vi "数据写入database.vi"(9 "data输入":T2) -> (1 "error out":errorcluster)   [LabVIEW 2016, in "斯坦道CODMn.lvlib"]
uses:
  <vilib>/Utility/error.llb/DialogType.ctl
panel:
  out "输出簇":T1
  in  "error in (no error)":errorcluster
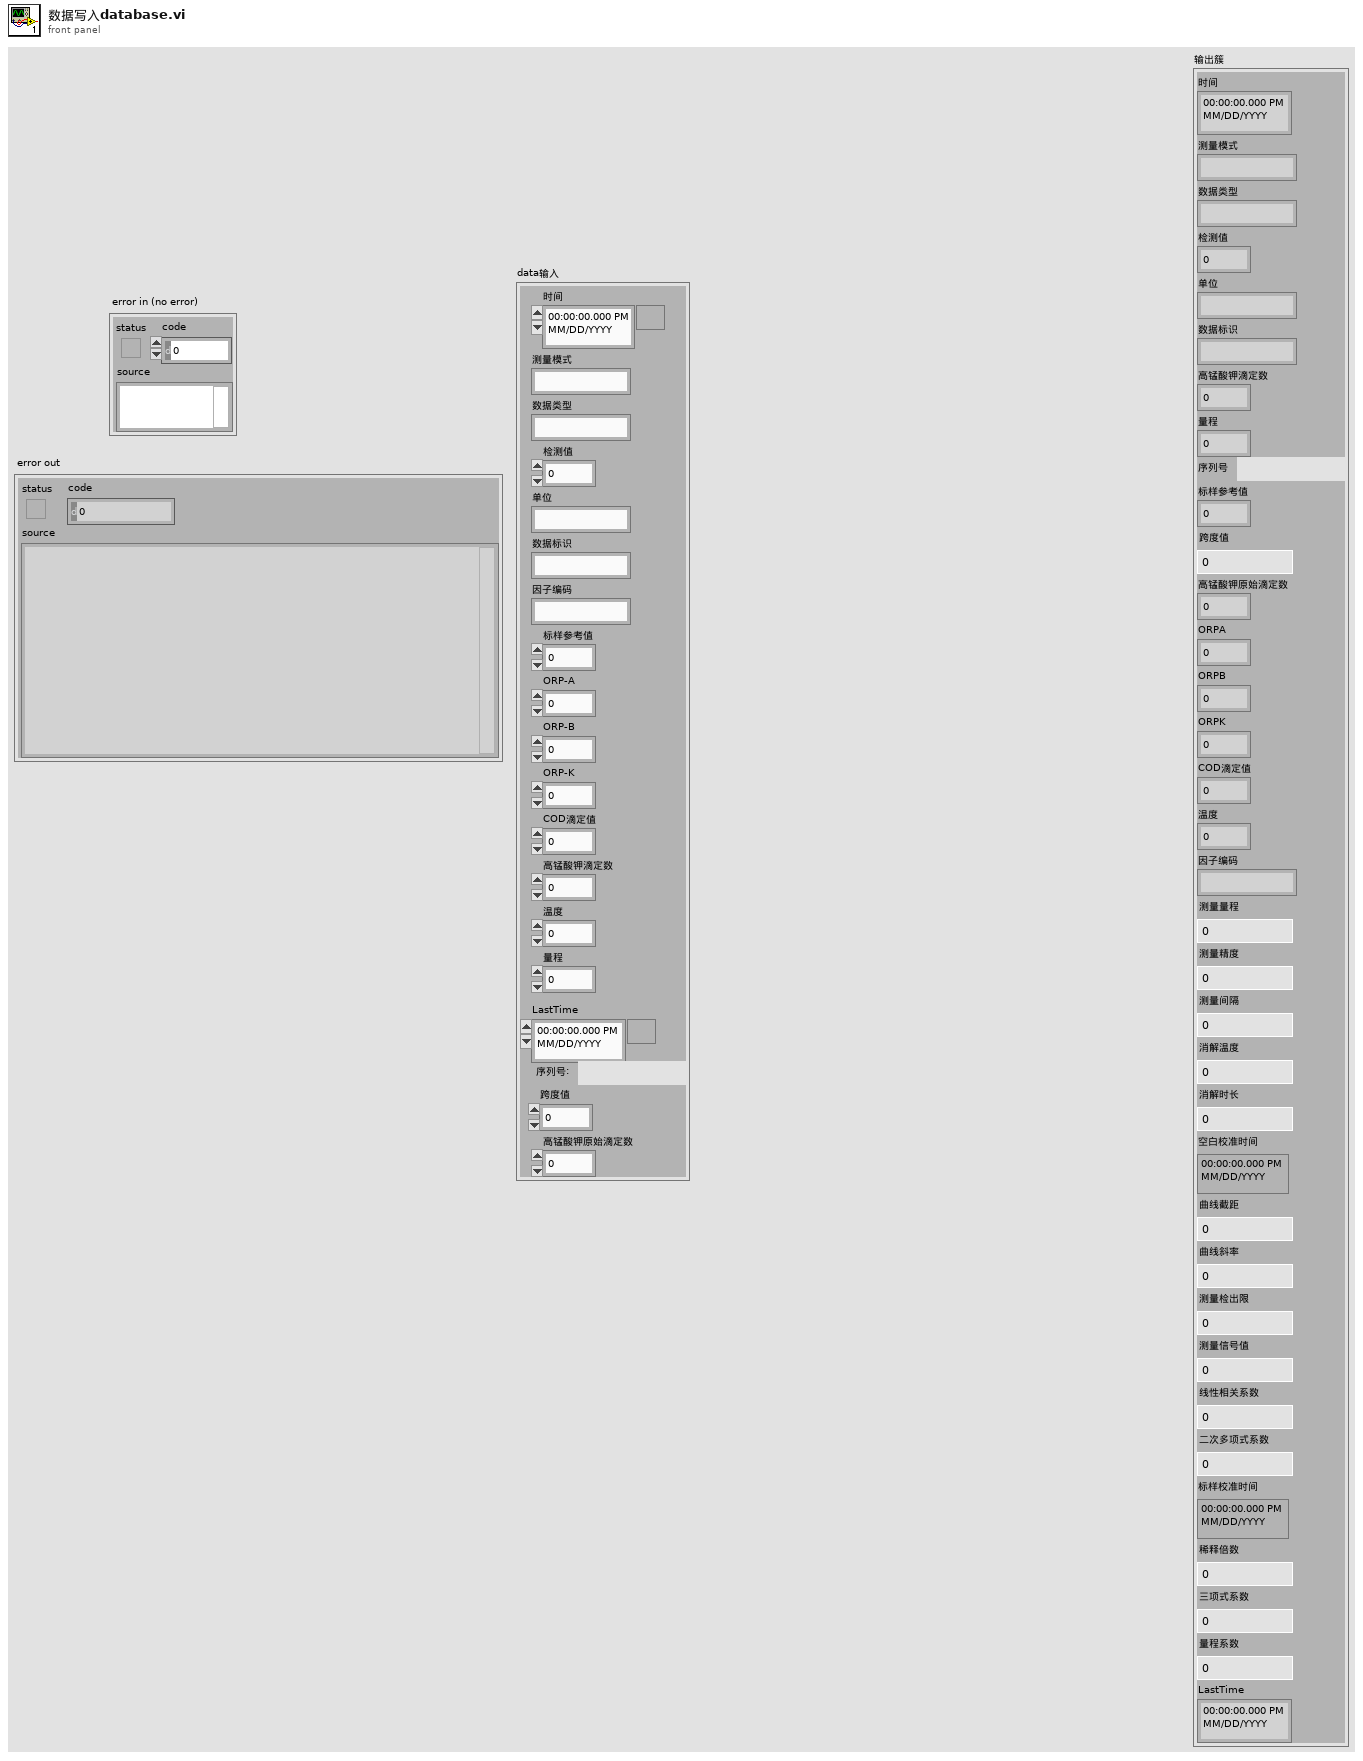
[diagram p1: front panel]
types:
  T1 = typedef "PLC版 CODMn字段定义.ctl" = cluster{"时间":timestamp, "测量模式":string, "数据类型":string, "检测值":sgl, "单位":string, "数据标识":string, "高锰酸钾滴定数":sgl, "量程":sgl, "序列号":string, "标样参考值":sgl, "跨度值":sgl, "高锰酸钾原始滴定数":sgl, "ORPA":sgl, "ORPB":sgl, "ORPK":sgl, "COD滴定值":sgl, "温度":sgl, "因子编码":string, "测量量程":sgl, "测量精度":sgl, "测量间隔":sgl, "消解温度":sgl, "消解时长":sgl, "空白校准时间":timestamp, "曲线截距":sgl, "曲线斜率":sgl, "测量检出限":sgl, "测量信号值":sgl, "线性相关系数":sgl, "二次多项式系数":sgl, "标样校准时间":timestamp, "稀释倍数":sgl, "三项式系数":sgl, "量程系数":sgl, "LastTime":timestamp}
  T2 = cluster{"时间":timestamp, "测量模式":string, "数据类型":string, "检测值":sgl, "单位":string, "数据标识":string, "因子编码":string, "标样参考值":sgl, "ORP-A":sgl, "ORP-B":sgl, "ORP-K":sgl, "COD滴定值":sgl, "高锰酸钾滴定数":sgl, "温度":sgl, "量程":sgl, "LastTime":timestamp, "序列号:":string, "跨度值":sgl, "高锰酸钾原始滴定数":sgl}
  T3 = typedef "DialogType.ctl" = u16
  T4 = cluster{"测量量程":dbl, "测量精度":dbl, "测量间隔":dbl, "消解温度":dbl, "消解时长":dbl, "空白校准时间":timestamp, "曲线截距":dbl, "曲线斜率":dbl, "测量检出限":dbl, "测量信号值":dbl, "线性相关系数":dbl, "二次多项式系数":dbl, "标样校准时间":timestamp, "稀释倍数":dbl, "三项式系数":dbl, "空白标定系数":dbl, "量程系数":dbl, "F0/ORPA":dbl, "F1/ORPB":dbl, "F2/ORPK":dbl, "F3":dbl, "F4":dbl, "F5":dbl, "F6":dbl, "F7":dbl, "X0/滴定数":dbl, "量程":dbl}
  T5 = typedef "数据库类型.ctl" = enum16{"Access", "SQLite"}
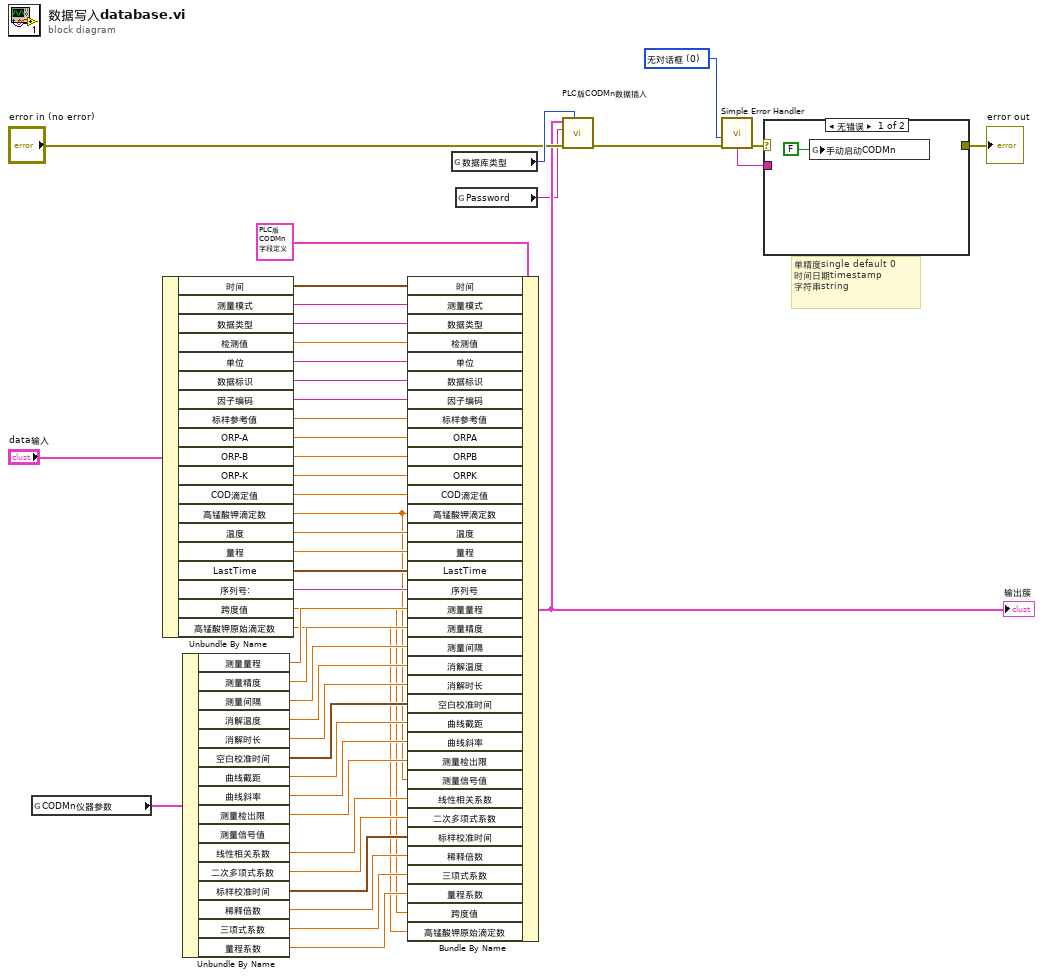
[diagram p0: block diagram]
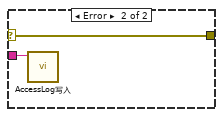
[diagram p2: hidden frame]
diagram:
  w46 = T3 0 items=["无对话框", "确定信息", "继续或停止信息", "确定信息＋警告", "继续/停止+警告"] ("type of dialog (OK msg:1)")
  # "单精度single default 0\n时间日期timestamp\n字符串string"
  n1 = global read "CODMn断电保存全局变量.vi" "CODMn仪器参数"() -> (w25:T4)
  n2 = Unbundle By Name("data输入") -> ("时间"=w41:timestamp, "测量模式"=w40:string, "数据类型"=w39:string, "检测值"=w38:sgl, "单位"=w37:string, "数据标识"=w36:string, "因子编码"=w35:string, "标样参考值"=w34:sgl, "ORP-A"=w33:sgl, "ORP-B"=w32:sgl, "ORP-K"=w31:sgl, "COD滴定值"=w30:sgl, "高锰酸钾滴定数"=w8:sgl, "温度"=w29:sgl, "量程"=w28:sgl, "LastTime"=w27:timestamp, "序列号:"=w26:string, "跨度值"=w9:sgl, "高锰酸钾原始滴定数"=w2:sgl)
  n3 = Unbundle By Name(w25) -> ("测量量程"=w24:dbl, "测量精度"=w23:dbl, "测量间隔"=w22:dbl, "消解温度"=w21:dbl, "消解时长"=w20:dbl, "空白校准时间"=w19:timestamp, "曲线截距"=w18:dbl, "曲线斜率"=w17:dbl, "测量检出限"=w16:dbl, "线性相关系数"=w15:dbl, "二次多项式系数"=w14:dbl, "标样校准时间"=w13:timestamp, "稀释倍数"=w12:dbl, "三项式系数"=w11:dbl, "量程系数"=w10:dbl)  [unwired: 1 out]
  n4 = Bundle By Name(cluster=T1 {"时间"=timestamp(0 s since 1904-01-01), "测量模式"="水样测试", "数据类型"="N", "检测值"=0.0, "单位"="mg/L", "数据标识"="N", "高锰酸钾滴定数"=0.0, "量程"=0.0, "序列号"="", "标样参考值"=0.0, "跨度值"=0.0, "高锰酸钾原始滴定数"=0.0, "ORPA"=0.0, "ORPB"=0.0, "ORPK"=0.0, "COD滴定值"=0.0, "温度"=0.0, "因子编码"="", "测量量程"=0.0, "测量精度"=0.0, "测量间隔"=0.0, "消解温度"=0.0, "消解时长"=0.0, "空白校准时间"=timestamp(0 s since 1904-01-01), "曲线截距"=0.0, "曲线斜率"=0.0, "测量检出限"=0.0, "测量信号值"=0.0, "线性相关系数"=0.0, "二次多项式系数"=0.0, "标样校准时间"=timestamp(0 s since 1904-01-01), "稀释倍数"=0.0, "三项式系数"=0.0, "量程系数"=0.0, "LastTime"=timestamp(0 s since 1904-01-01)} ("data"), "时间"=w41, "测量模式"=w40, "数据类型"=w39, "检测值"=w38, "单位"=w37, "数据标识"=w36, "因子编码"=w35, "标样参考值"=w34, "ORPA"=w33, "ORPB"=w32, "ORPK"=w31, "COD滴定值"=w30, "高锰酸钾滴定数"=w8, "温度"=w29, "量程"=w28, "LastTime"=w27, "序列号"=w26, "测量量程"=w24, "测量精度"=w23, "测量间隔"=w22, "消解温度"=w21, "消解时长"=w20, "空白校准时间"=w19, "曲线截距"=w18, "曲线斜率"=w17, "测量检出限"=w16, "测量信号值"=w8, "线性相关系数"=w15, "二次多项式系数"=w14, "标样校准时间"=w13, "稀释倍数"=w12, "三项式系数"=w11, "量程系数"=w10, "跨度值"=w9, "高锰酸钾原始滴定数"=w2) -> (w3:T1)
  "输出簇" <- w3
  n5 = global read "CODMn断电保存全局变量.vi" "数据库类型"() -> (w7:T5)
  n6 = global read "CODMn断电保存全局变量.vi" "Password"() -> (w1:string)
  n7 = call "PLC版CODMn数据插入.vi"("data"=w3, "Password"=w1, "错误输入（无错误）"="error in (no error)", "数据库类型"=w7) -> ("错误输出"=w5:errorcluster)  [unwired: 6 in]
  n8 = call <vilib>:"Simple Error Handler.vi"("type of dialog (OK msg:1)"=w46, "error in (no error)"=w5) -> ("error out"=w45:errorcluster, "message"=w43:string)  [unwired: 3 in, 3 out]
  n9 = case shown="无错误" w45 {
    selector: w45 -> [_ w48]
    tunnel: [_ w48] -> w44
    tunnel: w43 -> [_ w49]
    frame No Error {
      n10 = global write "CODMN外部API.vi" "手动启动CODMn"(FALSE ("手动启动CODMn")) -> ()
    }
    frame Error {
      n11 = call "AccessLog写入.vi"("Log"=w49) -> ()  [unwired: 11 in]
    }
  }
  "error out" <- w44
